vi "DownloadAnalysisData.vi"(8 "ErrorIn":errorcluster, 11 "QueuesIn":T1) -> (0 "ErrorOut":errorcluster)   [LabVIEW 2019]
uses:
  utilities/Queues.ctl
  GUIVIs/GUIOutput.ctl
  MobileAnalyzer/mainVIs/analyzeAccelerationDataVIs/AccelerationDataFrames.ctl
  MobileAnalyzer/mainVIs/analyzeAccelerationDataVIs/AnalyzedVibrationsData.ctl
  MobileAnalyzer/mainVIs/analyzeAccelerationDataVIs/calculateFaultIndicatorsVIs/FaultDetections.ctl
  MobileAnalyzer/mainVIs/analyzeAccelerationDataVIs/calculateFaultIndicatorsVIs/ParameterFaultDetection.ctl
  MobileAnalyzer/mainVIs/analyzeAccelerationDataVIs/calculateFaultIndicatorsVIs/FaultParameter.ctl
  MobileAnalyzer/mainVIs/analyzeAccelerationDataVIs/calculateFaultIndicatorsVIs/FrequencyFaultDetection.ctl
  masterVIs/Command.ctl
  MobileAnalyzer/mainVIs/TDMSmanagerVIs/TDMSAnalyzerData.ctl
  MobileAnalyzer/mainVIs/TDMSmanagerVIs/TDMSAnalyzerDataType.ctl
  masterVIs/Thread.ctl
  masterVIs/CommandQueuesAction.ctl
panel:
  out "Pobieranie":bool
  in  "DataDir":path=path "D:/studia/Praca Magisterska/VibrationDiagnosis/SavedData"
  in  "Delete all data":bool
  in  "Download data":bool
  in  "Close":bool
  # "Wybierz folder na dane z analizatora:"
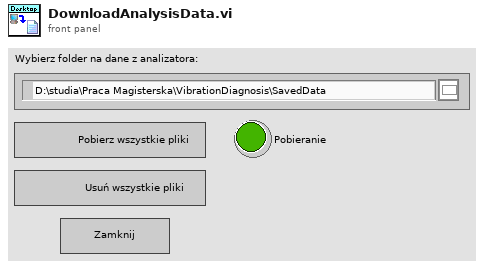
[diagram p1: front panel]
types:
  T1 = typedef "Queues.ctl" = cluster{"GUIOutput":refnum<queue>, "DataToSave":refnum<queue>, "AnalyzedVibrationsData":refnum<queue>, "Command":refnum<queue>, "TDMSAnalyzerData":refnum<queue>}
  T2 = typedef "TDMSAnalyzerDataType.ctl" = enum16{"FileDataStart", "FileGroup", "FileDataStop", "NewFile", "EndOfFile"}
  T3 = typedef "Command.ctl" = enum16{"None", "Connect", "Start", "Stop", "RestartAnalyzer", "Exit", "OpenDataFile", "CanBegin", "FileToSaveSettings", "AnalyzerSettings", "DownloadDataDialog", "DownloadData", "DeleteData"}
  T4 = typedef "CommandQueuesAction.ctl" = enum16{"Initialize", "Set", "Get", "ReleaseAll"}
  T5 = enum16{"open", "open or create", "create or replace", "create", "open (read-only)"}
  T6 = typedef "Thread.ctl" = enum16{"GUI", "communicateWithAnalyzer", "saveDataToTDMS"}
  T7 = typedef "TDMSAnalyzerData.ctl" = cluster{"TDMSAnalyzerDataType":T2, "group name out":string, "channel name(s) out":string[], "data":waveform(dbl)[], "File name":string}
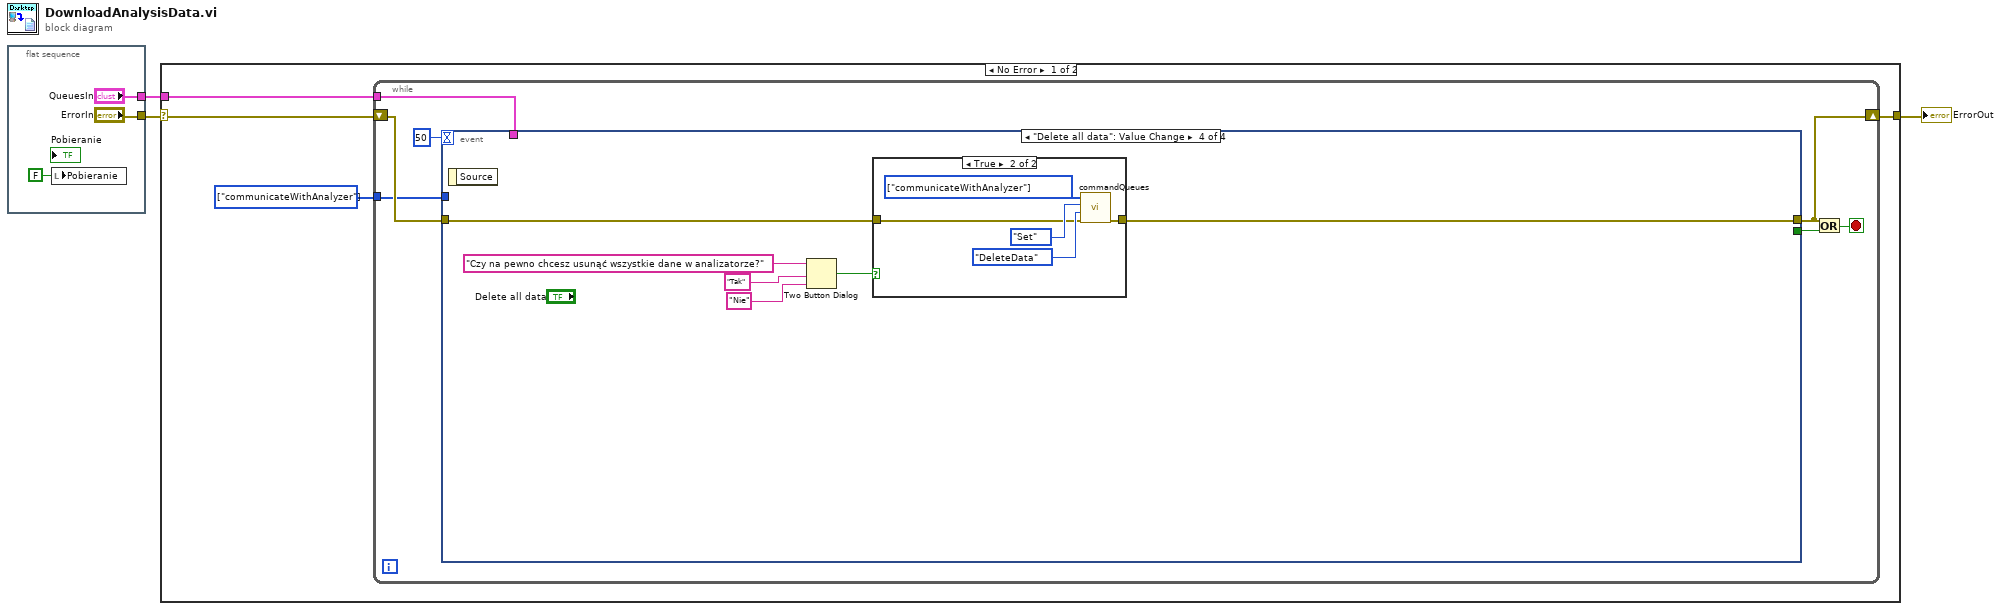
[diagram p0: block diagram]
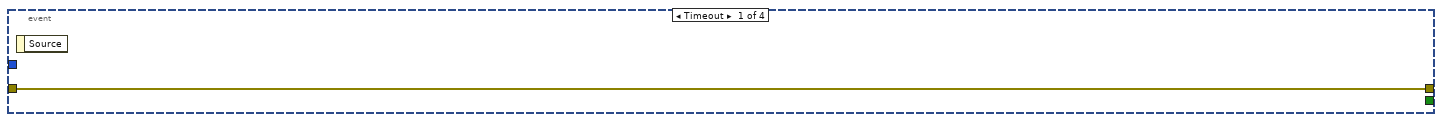
[diagram p2: hidden frame]
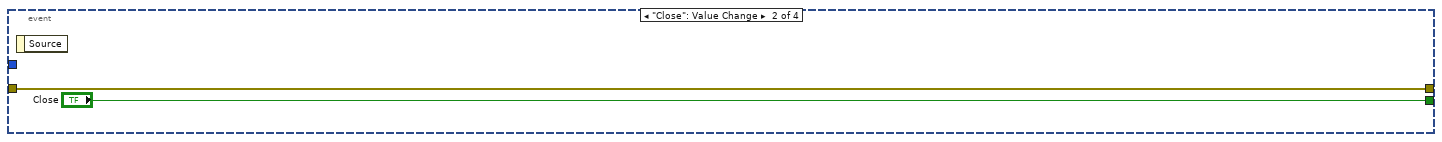
[diagram p3: hidden frame]
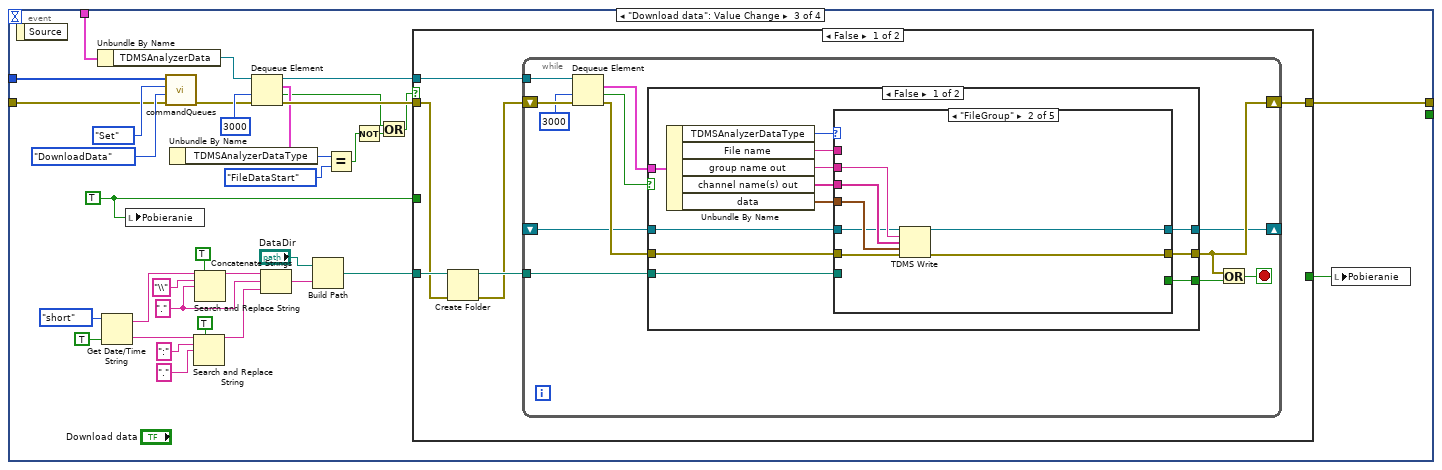
[diagram p4: hidden frame]
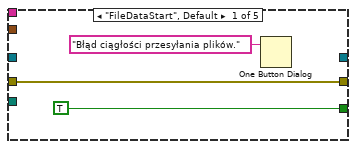
[diagram p5: hidden frame]
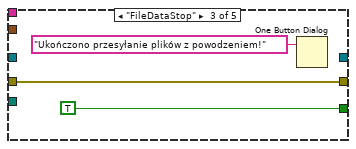
[diagram p6: hidden frame]
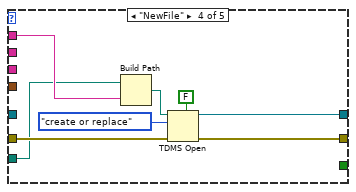
[diagram p7: hidden frame]
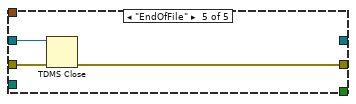
[diagram p8: hidden frame]
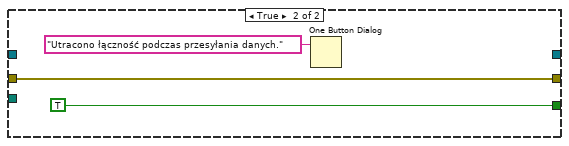
[diagram p9: hidden frame]
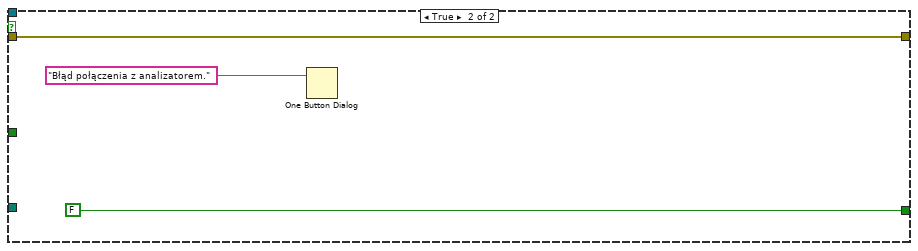
[diagram p10: hidden frame]
diagram:
  n1 = flat-sequence {
    tunnel: ["ErrorIn"] -> w3
    tunnel: ["QueuesIn"] -> w1
    frame #0 {
      n2 = local write "Pobieranie"(FALSE ("Pobieranie")) -> ()
    }
  }
  n3 = case shown="No Error" w3 {
    selector: w3 -> [w10 w128]
    tunnel: [w9 w128] -> w2
    tunnel: w1 -> [w7 _]
    frame No Error {
      w8 = T6[] [enum."communicateWithAnalyzer"] items=["GUI", "communicateWithAnalyzer", "saveDataToTDMS"] ("Threads")
      n4 = while {
        shift-right: [w12] -> w9
        shift-left: w10 -> [w14]
        tunnel: w8 -> [w13]
        tunnel: w7 -> [w11]
        stop <- w17 stop-if-true
        n5 = event shown="[3] \"Delete all data\": Value Change" {
          selector: _ -> [_ _ _ _]
          dyn-events: _ -> [_ _ _ _]
          timeout: 50 -> [_ _ _ _]
          tunnel: [_ "Close" _ _] -> w15
          tunnel: w14 -> [w18 w19 w52 w121]
          tunnel: w13 -> [_ _ w54 _]
          tunnel: [w18 w19 w44 w120] -> w12
          tunnel: w11 -> [_ _ w48 _]
          event Timeout {
            n6 = event-data() -> ()  [unwired: 1 in, 1 out]
          }
          event "Close": Value Change {
            n7 = event-data() -> ()  [unwired: 1 in, 1 out]
          }
          event "Download data": Value Change {
            w29 = "." ("replace string (\"\")")
            w51 = TRUE ("Pobieranie")
            n8 = event-data() -> ()  [unwired: 1 in, 1 out]
            n9 = Unbundle By Name(w48) -> ("TDMSAnalyzerData"=w50:refnum<queue>)
            n10 = Get Date/Time String(date format (0)=enum16{"short", "long", "abbreviated"}."short", want seconds? (F)=TRUE) -> (date string=w32:string, time string=w24:string)  [unwired: 1 in]
            n11 = local write "Pobieranie"(w51) -> ()
            n12 = call "commandQueues.vi"("ErrorIn"=w52, "CommandIn"=Command."DownloadData", "CommandQueuesAction"=CommandQueuesAction."Set", "Threads"=w54) -> ("ErrorOut"=w47:errorcluster)  [unwired: 6 in, 1 out]
            n13 = Search and Replace String(replace all?=TRUE ("replace all? (F)"), input string=w24, search string=":", replace string="." ("replace string (\"\")")) -> (result string=w21:string)  [unwired: 4 in, 3 out]
            n14 = Search and Replace String(replace all?=TRUE ("replace all? (F)"), input string=w32, search string="\\", replace string=w29) -> (result string=w30:string)  [unwired: 4 in, 3 out]
            n15 = Dequeue Element(queue=w50, timeout in ms (-1)=3000, error in (no error)=w47) -> (queue out=w45:refnum<queue>, element=w42:T7, timed out?=w38:bool, error out=w46:errorcluster)
            n16 = Unbundle By Name(w42) -> ("TDMSAnalyzerDataType"=w41:T2)
            n17 = Concatenate Strings(w30, w29, w21) -> (w28:string)
            n18 = Build Path(base path="DataDir", name or relative path=w28) -> (appended path=w26:path)
            n19 = Equal?(x=w41, y=TDMSAnalyzerDataType."FileDataStart") -> (x = y?=w39:bool)
            n20 = Not(x=w39) -> (.not. x?=w37:bool)
            n21 = Or(x=w38, y=w37) -> (x .or. y?=w36:bool)
            n22 = case shown="False" w36 {
              tunnel: w51 -> [_ _]
              tunnel: w46 -> [w57 w114]
              tunnel: w45 -> [w61 _]
              tunnel: [w60 w114] -> w44
              tunnel: [_ FALSE ("Close")] -> w43
              tunnel: w26 -> [w59 _]
              frame False {
                n23 = Create Folder(path (use dialog)=w59, error in=w57) -> (created path=w58:path, error out=w56:errorcluster)  [unwired: 1 in, 1 out]
                n24 = while {
                  tunnel: w61 -> [w71]
                  shift-right: [w67] -> w60
                  shift-left: w56 -> [w73]
                  shift-right: [w63] -> _
                  shift-left: _ -> [w64]
                  tunnel: w58 -> [w62]
                  stop <- w65 stop-if-true
                  n25 = Dequeue Element(queue=w71, timeout in ms (-1)=3000, error in (no error)=w73) -> (element=w70:T7, timed out?=w69:bool, error out=w68:errorcluster)  [unwired: 1 out]
                  n26 = case shown="False" w69 {
                    tunnel: w70 -> [w85 _]
                    tunnel: w68 -> [w79 w112]
                    tunnel: [w78 w112] -> w67
                    tunnel: [w77 TRUE] -> w66
                    tunnel: w64 -> [w76 _]
                    tunnel: [w75 _] -> w63
                    tunnel: w62 -> [w74 _]
                    frame False {
                      n27 = Unbundle By Name(w85) -> ("TDMSAnalyzerDataType"=w84:T2, "File name"=w83:string, "group name out"=w82:string, "channel name(s) out"=w81:string[], "data"=w80:waveform(dbl)[])
                      n28 = case shown="\"FileGroup\"" w84 {
                        tunnel: w83 -> [_ _ _ w103 _]
                        tunnel: w82 -> [_ w95 _ _ _]
                        tunnel: w81 -> [_ w94 _ _ _]
                        tunnel: w80 -> [_ w93 _ _ _]
                        tunnel: w79 -> [w87 w90 w98 w102 w108]
                        tunnel: [w87 w89 w98 w101 w107] -> w78
                        tunnel: [TRUE _ TRUE _ _] -> w77
                        tunnel: w76 -> [_ w91 _ _ w109]
                        tunnel: [_ w92 _ w100 _] -> w75
                        tunnel: w74 -> [_ _ _ w99 _]
                        frame "FileDataStart", Default {
                          n29 = One Button Dialog(message="Błąd ciągłości przesyłania plików.") -> ()  [unwired: 1 in, 1 out]
                        }
                        frame "FileGroup" {
                          n30 = TDMS Write(0:w91, 5:w95, 7:w94, 9:w93, 11:w90) -> (4:w92:refnum<k34>, 15:w89:errorcluster)  [unwired: 1 in, 2 out]
                        }
                        frame "FileDataStop" {
                          n31 = One Button Dialog(message="Ukończono przesyłanie plików z powodzeniem!") -> ()  [unwired: 1 in, 1 out]
                        }
                        frame "NewFile" {
                          n32 = Build Path(base path=w99, name or relative path=w103) -> (appended path=w106:path)
                          n33 = TDMS Open(5:FALSE ("create index file? (T)"), 8:w102, 10:T5."create or replace" ("operation (0:open)"), 11:w106) -> (0:w101:errorcluster, 3:w100:refnum<k34>)  [unwired: 3 in]
                        }
                        frame "EndOfFile" {
                          n34 = TDMS Close(8:w108, 11:w109) -> (0:w107:errorcluster)  [unwired: 1 out]
                        }
                      }
                    }
                    frame True {
                      n35 = One Button Dialog(message="Utracono łączność podczas przesyłania danych.") -> ()  [unwired: 1 in, 1 out]
                    }
                  }
                  n36 = Or(x=w67, y=w66) -> (x .or. y?=w65:bool)
                }
              }
              frame True {
                n37 = One Button Dialog(message="Błąd połączenia z analizatorem.") -> ()  [unwired: 1 in, 1 out]
              }
            }
            n38 = local write "Pobieranie"(w43) -> ()
          }
          event "Delete all data": Value Change {
            n39 = event-data() -> ()  [unwired: 1 in, 1 out]
            n40 = Two Button Dialog(message="Czy na pewno chcesz usunąć wszystkie dane w analizatorze?", 1:"Nie" ("F button name (\"Cancel\")"), 2:"Tak" ("T button name (\"OK\")")) -> (T button?=w116:bool)
            n41 = case shown="True" w116 {
              tunnel: w121 -> [w122 w125]
              tunnel: [w122 w124] -> w120
              frame False {
              }
              frame True {
                w123 = T6[] [enum."communicateWithAnalyzer"] items=["GUI", "communicateWithAnalyzer", "saveDataToTDMS"] ("Threads")
                n42 = call "commandQueues.vi"("ErrorIn"=w125, "CommandIn"=Command."DeleteData", "CommandQueuesAction"=CommandQueuesAction."Set", "Threads"=w123) -> ("ErrorOut"=w124:errorcluster)  [unwired: 6 in, 1 out]
              }
            }
          }
        }
        n43 = Or(x=w12, y=w15) -> (x .or. y?=w17:bool)
      }
    }
    frame Error {
    }
  }
  "ErrorOut" <- w2
